vi "Calculate PRF.vi"(1 "PRF":dbl) -> (0 "PRF Array":dbl[](array[numeric]))   [LabVIEW 2016]
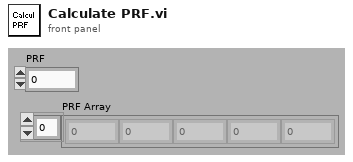
[diagram p1: front panel]
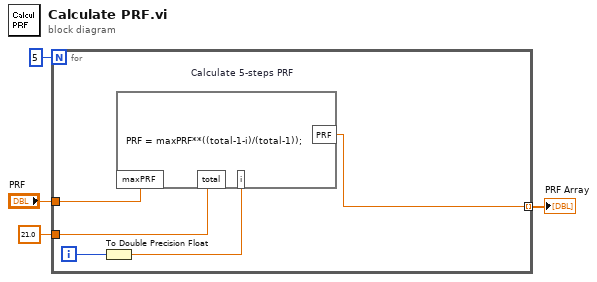
[diagram p0: block diagram]
diagram:
  n1 = for {
    N: 5 -> [_]
    tunnel: "PRF" -> [w9]
    tunnel: 21.0 ("input variable") -> [w6]
    tunnel: [w5] -> w2 mode=indexing
    i -> [w7]
    n2 = To Double Precision Float(number=w7) -> (double precision float=w8:dbl)
    n3 = formula code="PRF = maxPRF**((total-1-i)/(total-1));" "Calculate 5-steps PRF"("total"=w6, "maxPRF"=w9, "i"=w8) -> ("PRF"=w5:dbl)
  }
  "PRF Array" <- w2
